vi "LS330_ReadDate.vi"(8 "error in":errorcluster, 11 "refnum":refnum<file>) -> (0 "error out":errorcluster, 2 "Date":timestamp, 3 "refnum 2":refnum<file>)   [LabVIEW 2021]
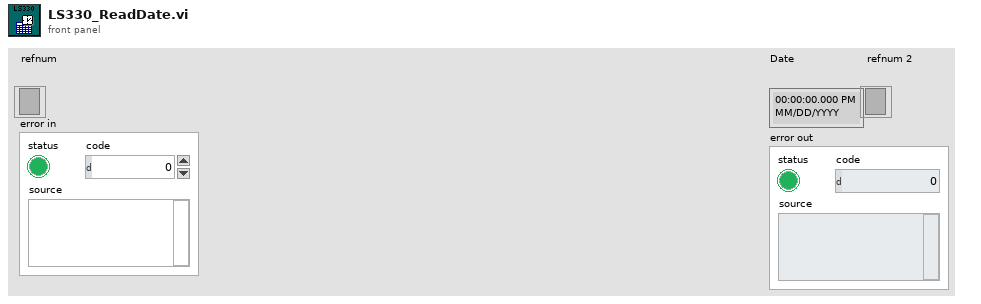
[diagram p1: front panel]
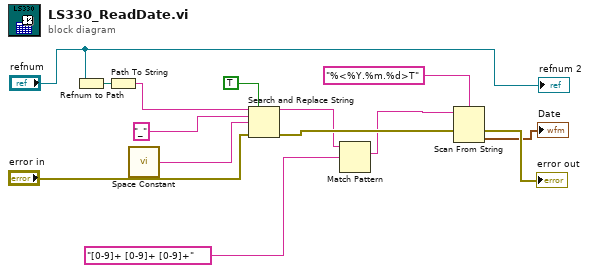
[diagram p0: block diagram]
diagram:
  n1 = Refnum to Path(1:"refnum") -> (0:w14:path)
  n2 = Path To String(path=w14) -> (string=w12:string)
  n3 = call <vilib>:"Space Constant.vi"() -> ("String"=w9:string)
  n4 = Search and Replace String(replace all?=TRUE ("replace all? (F)"), input string=w12, search string="_", replace string=w9, error in="error in") -> (result string=w3:string, error out=w8:errorcluster)  [unwired: 3 in, 2 out]
  n5 = Match Pattern(string=w3, regular expression="[0-9]+ [0-9]+ [0-9]+") -> (match substring=w1:string)  [unwired: 1 in, 3 out]
  n6 = Scan From String(format string="%<%Y.%m.%d>T", input string=w1, error in=w8) -> (error out=→"error out":errorcluster, output 1=→"Date":timestamp)  [unwired: 2 in, 2 out]
  "refnum 2" <- "refnum"
